vi "E_error_check.vi"(4 "Error in":errorcluster) -> (0 "code":i32, 1 "Error out":errorcluster, 2 "Fatal Error":bool)   [LabVIEW 2013]
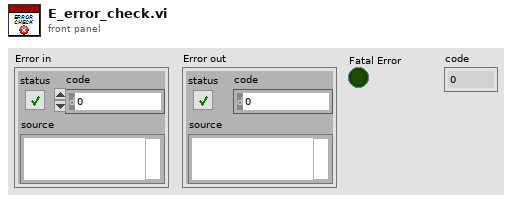
[diagram p1: front panel]
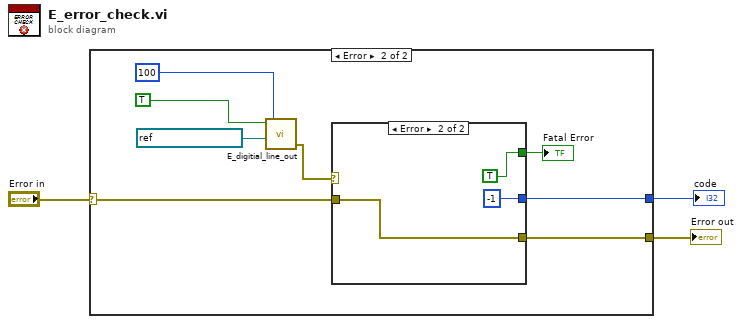
[diagram p0: block diagram]
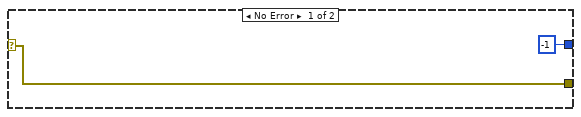
[diagram p2: hidden frame]
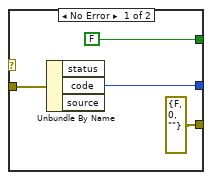
[diagram p3: hidden frame]
diagram:
  n1 = case shown="Error" "Error in" {
    selector: "Error in" -> [w5 w8]
    tunnel: [w5 w7] -> w2
    tunnel: [-1 ("code") w6] -> w1
    frame No Error {
    }
    frame Error {
      n2 = call "E_digitial_line_out.vi"("task/channels in"=refnum<k21> "ErrorCheckOut", "milliseconds to wait"=u32 100, "Boolean"=TRUE) -> ("error out"=w10:errorcluster)  [unwired: 3 in]
      n3 = case shown="Error" w10 {
        tunnel: [FALSE TRUE] -> w9
        tunnel: [errorcluster {"status"=FALSE, "code"=0, "source"=""} ("error IO") w19] -> w7
        tunnel: w8 -> [w16 w19]
        tunnel: [w14 -1 ("code")] -> w6
        frame No Error {
          n4 = Unbundle By Name(w16) -> ("code"=w14:i32)  [unwired: 2 out]
        }
        frame Error {
        }
      }
      "Fatal Error" <- w9
    }
  }
  "Error out" <- w2
  "code" <- w1
